vi "TagContainer-TestMain.vi"() -> ()   [LabVIEW 2017]
uses:
  a1ae43e1-b2e0-48b2-b5bf-09d8c6337ec0.vi
  5d4c14d8-f2b2-4cd0-9f9f-81160b0f88f4.vi
  69a5f5dc-289e-4520-a43d-4a6e53800127.vi
  f6a41f1a-46ba-40d5-b8b9-4f6d9d3cd2d0.vi
  b9594d6d-a8e1-4e69-b527-0d31d87043e6.vi
  TagContainer/_Support/_NameCacher.vi
  TagContainer/_Support/_datatypeChecker.vi
  TagContainer/_Support/_Ref To DVR.vi
  TagContainer/API/TagContainer-ChangeDetector.vi/4615f950-5bb4-4f5c-be7d-266d36556fe4.vi
  <vilib>/Utility/Data Type/Get Type Information.vi
  <vilib>/Utility/error.llb/Trim Whitespace.vi
  TagContainer/TagContainer.lvlib
panel:
  out "TEst":cluster{"Numeric":i32, "String":string}
  out "changed?":bool[](array[boolean])
  in  "Reject New Tag(F)":bool=TRUE
  out "should be datatype error":errorcluster
  out "should be no tag error":errorcluster
  out "Raw name":string
  in  "Type":cluster{"Numeric":i32, "String":string}
  in  "Stop":bool
  out "Value":cluster{"Numeric":i32, "String":string}
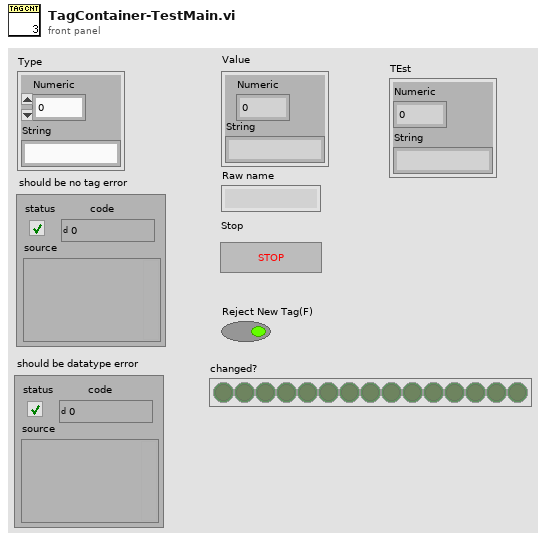
[diagram p1: front panel]
types:
  T1 = typedef "TagContainer.lvlib/TagContainer.ctl" = refnum<k1>
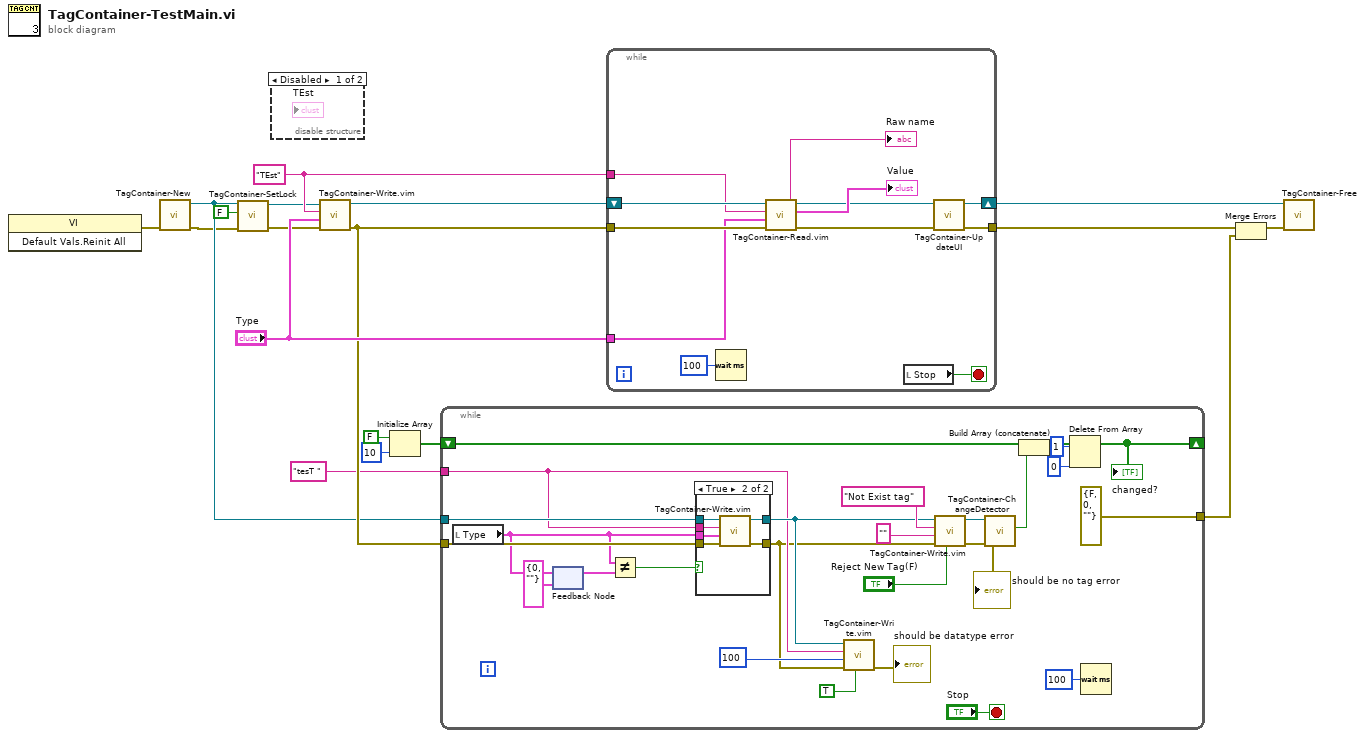
[diagram p0: block diagram]
diagram:
  w14 = "TEst" ("name")
  n1 = invoke class="VI" method="Default Vals.Reinit All"() -> (error out=w10:errorcluster)  [unwired: 3 in, 2 out]
  n2 = call "TagContainer-New.vi"("error in (no error)"=w10) -> ("error out"=w4:errorcluster, "TagContainer"=w5:T1)  [unwired: 9 in]
  n3 = call "TagContainer-SetLock.vi"("error in (no error)"=w4, "Lock?(T)"=FALSE, "TagContainer"=w5) -> ("error out"=w3:errorcluster, "TagContainer(dup)"=w2:T1)  [unwired: 7 in]
  n4 = disable-structure shown="Disabled" {
    frame Disabled {
    }
    frame Enabled {
    }
  }
  n5 = call "TagContainer-Write.vim"("error in (no error)"=w3, "Value"="Type", "name"=w14, "TagContainer"=w2) -> ("error out"=w13:errorcluster, "TagContainer(dup)"=w18:T1)  [unwired: 6 in]
  n6 = Initialize Array(FALSE, 10 ("dimension size")) -> (w6:bool[])
  n7 = while {
    tunnel: w5 -> [w42]
    tunnel: "tesT " ("name") -> [w34]
    tunnel: w13 -> [w41]
    tunnel: [errorcluster {"status"=FALSE, "code"=0, "source"=""} ("error out")] -> w11
    shift-right: [w25] -> _
    shift-left: w6 -> [w28]
    stop <- "Stop" stop-if-true
    n8 = local read "Type"() -> (w21:cluster{"Numeric":i32, "String":string})
    n9 = feedback-in #1(w21) -> ()
    n10 = feedback #1(cluster{"Numeric":i32, "String":string} {"Numeric"=0, "String"=""} ("Type")) -> (w20:cluster{"Numeric":i32, "String":string})
    n11 = Not Equal?(x=w21, y=w20) -> (x != y?=w22:bool)
    n12 = case shown="True" w22 {
      tunnel: w42 -> [w46 w52]
      tunnel: w41 -> [w45 w51]
      tunnel: [w46 w50] -> w35
      tunnel: w34 -> [_ w49]
      tunnel: [w45 w48] -> w32
      tunnel: w21 -> [_ w47]
      frame False {
      }
      frame True {
        n13 = call "TagContainer-Write.vim"("error in (no error)"=w51, "Value"=w47, "name"=w49, "TagContainer"=w52) -> ("error out"=w48:errorcluster, "TagContainer(dup)"=w50:T1)  [unwired: 6 in]
      }
    }
    n14 = call "TagContainer-Write.vim"("Reject New Tag(F)"=TRUE, "error in (no error)"=w32, "Value"=u32 100 ("milliseconds to wait"), "name"=w34, "TagContainer"=w35) -> ("error out"=→"should be datatype error":errorcluster)  [unwired: 5 in, 1 out]
    n15 = call "TagContainer-Write.vim"("Reject New Tag(F)"="Reject New Tag(F)", "error in (no error)"=w32, "Value"="" ("name"), "name"="Not Exist tag", "TagContainer"=w35) -> ("error out"=→"should be no tag error":errorcluster, "TagContainer(dup)"=w29:T1)  [unwired: 5 in]
    n16 = call "TagContainer-ChangeDetector.vi"("TagContainer"=w29) -> ("Changed"=w27:bool)  [unwired: 8 in, 2 out]
    n17 = Build Array (concatenate)(w28, w27) -> (w26:bool[])
    n18 = Delete From Array(array=w26, length=1, index=0) -> (array with subset deleted=w25:bool[])  [unwired: 1 out]
    "changed?" <- w25
    n19 = Wait (ms)(milliseconds to wait=u32 100) -> ()  [unwired: 1 out]
  }
  n20 = while {
    tunnel: w14 -> [w62]
    tunnel: "Type" -> [w61]
    shift-right: [w53] -> w17
    shift-left: w18 -> [w64]
    tunnel: w13 -> [w63]
    tunnel: [w54] -> w16
    stop <- w59 stop-if-true
    n21 = Wait (ms)(milliseconds to wait=u32 100) -> ()  [unwired: 1 out]
    n22 = call "TagContainer-Read.vim"("error in (no error)"=w63, "Type"=w61, "name"=w62, "TagContainer"=w64) -> ("error out"=w55:errorcluster, "Value"=→"Value":cluster{"Numeric":i32, "String":string}, "TagContainer(dup)"=w56:T1, "Raw name"=→"Raw name":string)  [unwired: 2 in, 2 out]
    n23 = local read "Stop"() -> (w59:bool)
    n24 = call "TagContainer-UpdateUI.vi"("error in (no error)"=w55, "TagContainer"=w56) -> ("error out"=w54:errorcluster, "TagContainer(dup)"=w53:T1)  [unwired: 8 in]
  }
  n25 = Merge Errors(w16, w11) -> (w12:errorcluster)
  n26 = call "TagContainer-Free.vi"("error in (no error)"=w12, "TagContainer"=w17) -> ()  [unwired: 9 in, 1 out]
